vi "Pause Timer.vi"(8 "error in":errorcluster, 11 "Timer in":refnum<class "Timer.lvclass">) -> (0 "error out":errorcluster, 3 "Timer out":refnum<class "Timer.lvclass">)   [LabVIEW 2019, in "Timer.lvlib" / "Timer.lvclass"]
uses:
  Timer.lvclass
  Timer.lvclass/Timer.ctl
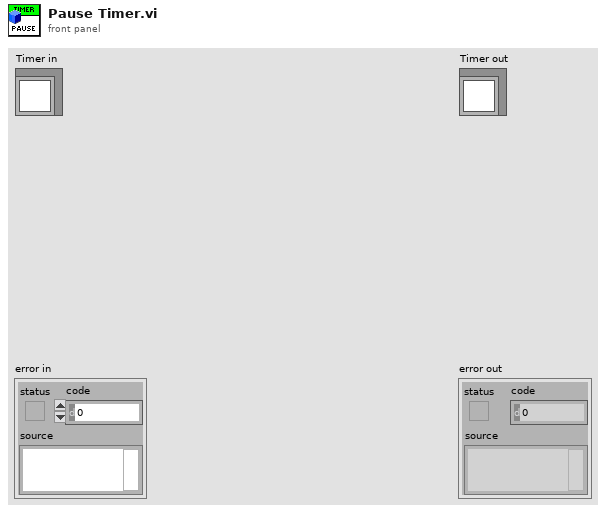
[diagram p1: front panel]
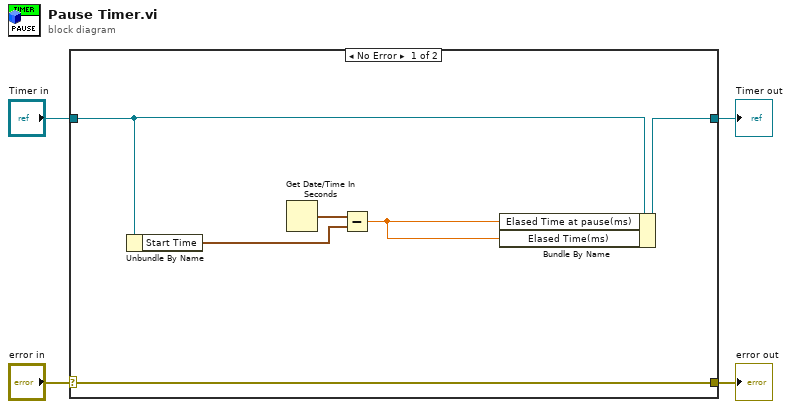
[diagram p0: block diagram]
diagram:
  n1 = case shown="No Error" "error in" {
    selector: "error in" -> [w10 w12]
    tunnel: [w10 w12] -> w3
    tunnel: [w7 w11] -> w1
    tunnel: "Timer in" -> [w8 w11]
    frame No Error {
      n2 = Unbundle By Name(w8) -> ("Start Time"=w9:timestamp)
      n3 = Get Date/Time In Seconds() -> (seconds since 1Jan1904=w6:timestamp)
      n4 = Subtract(x=w6, y=w9) -> (x-y=w5:dbl)
      n5 = Bundle By Name(cluster=w8, "Elased Time at pause(ms)"=w5, "Elased Time(ms)"=w5) -> (w7:refnum<class "Timer.lvclass">)
    }
    frame Error {
    }
  }
  "error out" <- w3
  "Timer out" <- w1
